vi "SwerveKinematics_ToTwist2dX.vi"(9 "WheelDeltas":T2[](array[typedef]) {"Angle"."SIN" format="%13.4f"; "Angle"."COS" format="%13.4f"; "Angle"."VALUE" format="%13.4f"}, 11 "in SWERVE_DRIVE_KINEMATICS":T4 {"SavedModuleStates"."Angle"."SIN" format="%13.4f"; "SavedModuleStates"."Angle"."COS" format="%13.4f"; "SavedModuleStates"."Angle"."VALUE" format="%13.4f"; "PrevCoR"."Y" format="%14.3f"; "PrevCoR"."X" format="%14.3f"; "Modules"."Y" format="%14.3f"; "Modules"."X" format="%14.3f"}) -> (1 "Error":bool, 3 "Twist2d":T1)   [LabVIEW 2019, in "Trajectory_Library.lvlib"]
doc: "Performs forward kinematics to return the resulting chassis state from the given module states. This method is often used for odometry -- determining the robot's position on the field using data from the real-world speed and angle of each module on the robot.\n\n\nParameters: \n - in Swerve Drive Kinematics - Swerve drive kinematics data structure\n - wheelDeltas - An array of the latest change in position of the modules (as a SwerveModulePosition type) as measured from respective encoders and gyros. The order of the swerve module states should be same as passed into the constructor of this class.\n\nReturns:\n - The resulting twist2d."
uses:
  Trajectory_Library.lvlib
  TypeDef/SWERVE_DRIVE_KINEMATICS.ctl
  <vilib>/Analysis/Matrix/Datatypes/RealMatrix.ctl
  TypeDef/TRANSLATION2D.ctl
  TypeDef/SWERVE_DRIVE_MODULE_STATE.ctl
  TypeDef/ROTATION2D.ctl
  TypeDef/SWERVE_DRIVE_MODULE_POSITION.ctl
  TypeDef/TWIST2D.ctl
  <vilib>/Analysis/Matrix/Numeric/Multiply/Multiply - RM,RM.vi
  <vilib>/Analysis/Matrix/NI_Matrix.lvlib
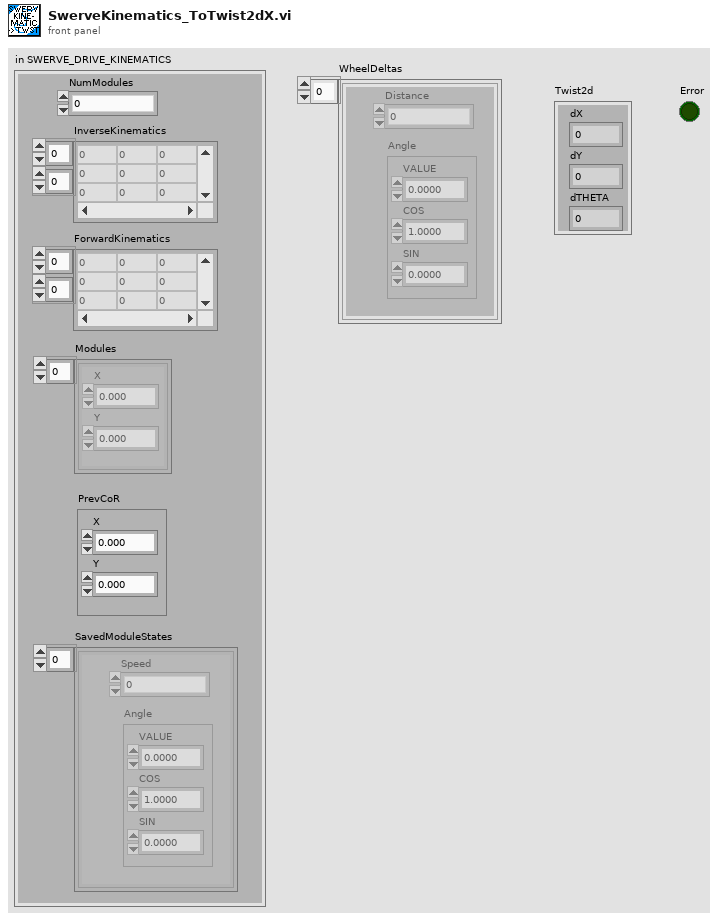
[diagram p1: front panel]
types:
  T1 = typedef "Trajectory_Library.lvlib/TWIST2D.ctl" = cluster{"dX":dbl, "dY":dbl, "dTHETA":dbl}
  T2 = typedef "Trajectory_Library.lvlib/SWERVE_DRIVE_MODULE_POSITION.ctl" = cluster{"Distance":dbl, "Angle":T3}
  T3 = typedef "Trajectory_Library.lvlib/ROTATION2D.ctl" = cluster{"VALUE":dbl, "COS":dbl, "SIN":dbl}
  T4 = typedef "Trajectory_Library.lvlib/SWERVE_DRIVE_KINEMATICS.ctl" = cluster{"NumModules":i32, "InverseKinematics":T5, "ForwardKinematics":T5, "Modules":T6[], "PrevCoR":T6, "SavedModuleStates":T7[]}
  T5 = typedef "NI_Matrix.lvlib/RealMatrix.ctl" = dbl[][]
  T6 = typedef "Trajectory_Library.lvlib/TRANSLATION2D.ctl" = cluster{"X":dbl, "Y":dbl}
  T7 = typedef "Trajectory_Library.lvlib/SWERVE_DRIVE_MODULE_STATE.ctl" = cluster{"Speed":dbl, "Angle":T3}
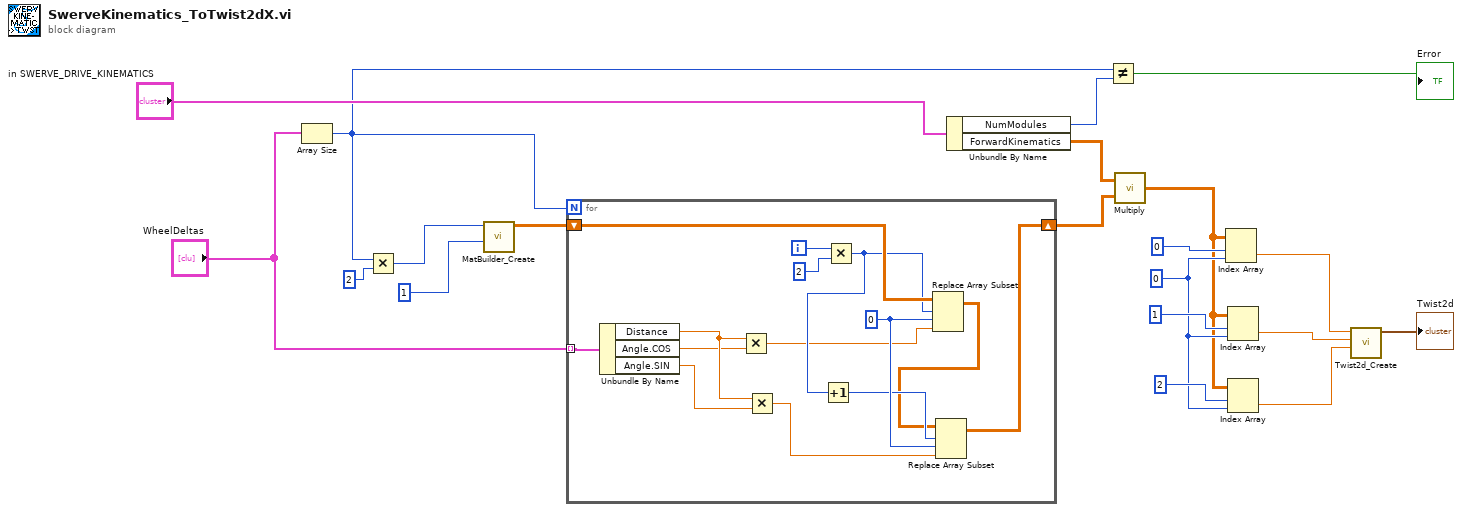
[diagram p0: block diagram]
diagram:
  w12 = 0 ("index (col)")
  n1 = Array Size(array="WheelDeltas") -> (size(s)=w2:i32)
  n2 = Multiply(x=w2, y=2) -> (x*y=w6:i32)
  n3 = call "MatBuilder_Create.vi"("Columns"=1 ("number of columns"), "Rows"=w6) -> ("output matrix"=w4:T5)  [unwired: 9 in]
  n4 = for {
    N: w2 -> [_]
    shift-right: [w26] -> w17
    shift-left: w4 -> [w34]
    tunnel: "WheelDeltas" -> [w28] mode=indexing
    i -> [w32]
    w33 = 0 ("disabled index (col)")
    n5 = Unbundle By Name(w28) -> ("Distance"=w25:dbl, "Angle.COS"=w24:dbl, "Angle.SIN"=w23:dbl)
    n6 = Multiply(x=w25, y=w24) -> (x*y=w22:dbl)
    n7 = Multiply(x=w25, y=w23) -> (x*y=w21:dbl)
    n8 = Multiply(x=w32, y=2) -> (x*y=w30:i32)
    n9 = Increment(x=w30) -> (x+1=w29:i32)
    n10 = Replace Array Subset(array=w34, new element=w22, index (row)=w30, index (col)=w33) -> (w27:T5)
    n11 = Replace Array Subset(array=w27, new element=w21, index (row)=w29, index (col)=w33) -> (w26:T5)
  }
  n12 = Unbundle By Name("in SWERVE_DRIVE_KINEMATICS") -> ("NumModules"=w3:i32, "ForwardKinematics"=w18:T5)
  n13 = Not Equal?(x=w2, y=w3) -> (x != y?=→"Error":bool)
  n14 = call-poly <vilib>:"Multiply.vi"("Real Matrix B"=w17, "Real Matrix A"=w18) -> ("A * B"=w11:T5)
  n15 = Index Array(array=w11, index (row)=0, index (col)=w12) -> (element=w10:dbl)
  n16 = Index Array(array=w11, index (row)=1, index (col)=w12) -> (element=w9:dbl)
  n17 = Index Array(array=w11, index (row)=2, index (col)=w12) -> (element=w8:dbl)
  n18 = call "Twist2d_Create.vi"("dTHETA"=w8, "dY"=w9, "dX"=w10) -> ("TWIST"=→"Twist2d":T1)  [unwired: 8 in]
